vi "Query Sys (To) Parameters (Mode).vi"(8 "error in (no error)":errorcluster, 11 "VISA resource name":refnum<visa-resource-name>) -> (0 "error out":errorcluster, 2 "Mode Parameters":T1={" Mode"=enum."Normal", "Burst #"=-1, "DC Off"=-1, "DC On"=-1, "Period"=nan} {"Period" format="%.6p"}, 3 "VISA resource name out":refnum<visa-resource-name>)   [LabVIEW 2013, in "Berkeley Nucleonics 500 Series.lvlib"]
doc: "This VI is used to read the mode configuration of the system timer (To)."
uses:
  Berkeley Nucleonics 500 Series.lvlib
panel:
  # "Burst"
  # "Duty\nCycle"
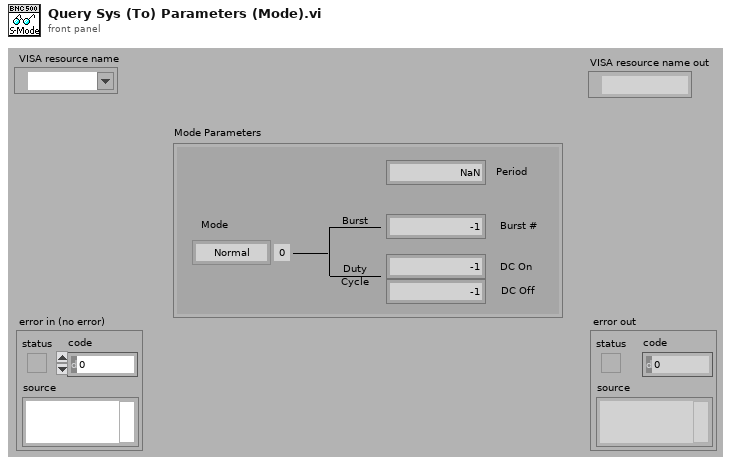
[diagram p1: front panel]
types:
  T1 = cluster{" Mode":enum16{"Normal", "Single", "Burst", "Duty Cycle"}, "Burst #":i32, "DC Off":i32, "DC On":i32, "Period":dbl}
  T2 = cluster{"Sys (To) Mode":enum16{"Normal", "Single", "Burst", "Duty Cycle"}, "Sys (To) Burst #":i32, "Sys (To) DC Off":i32, "Sys (To) DC On":i32, "Sys (To)  Period":dbl}
  T3 = enum16{"Normal", "Single", "Burst", "Duty Cycle"}
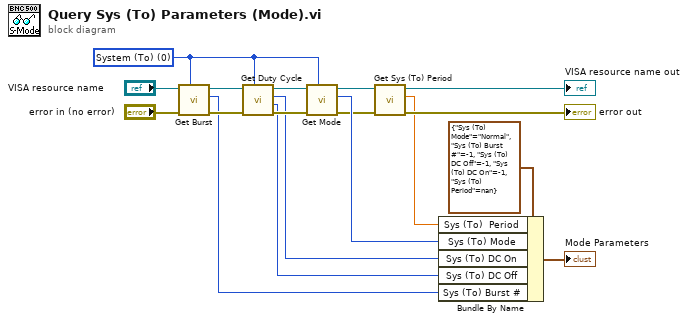
[diagram p0: block diagram]
diagram:
  w6 = 0 items=["System (To)", "Channel A", "Channel B", "Channel C", "Channel D", "Channel E", "Channel F", "Channel G", "Channel H"] ("Channel (1: Chan A)")
  n1 = call "Get Burst.vi"("Channel (1: Chan A)"=w6, "error in (no error)"="error in (no error)", "VISA resource name"="VISA resource name") -> ("error out"=w13:errorcluster, "Burst #"=w11:i32, "VISA resource name out"=w14:refnum<visa-resource-name>)  [unwired: 6 in]
  n2 = call "Get Duty Cycle.vi"("Channel (1: Chan A)"=w6, "error in (no error)"=w13, "VISA resource name"=w14) -> ("error out"=w16:errorcluster, "DC Off"=w10:i32, "DC On"=w9:i32, "VISA resource name out"=w15:refnum<visa-resource-name>)  [unwired: 5 in]
  n3 = call "Get Mode.vi"("Channel (1: Chan A)"=w6, "error in (no error)"=w16, "VISA resource name"=w15) -> ("error out"=w5:errorcluster, "Mode"=w12:T3, "VISA resource name out"=w3:refnum<visa-resource-name>)  [unwired: 6 in]
  n4 = call "Get Sys (To) Period.vi"("error in (no error)"=w5, "VISA resource name"=w3) -> ("error out"=→"error out":errorcluster, "Period"=w1:dbl, "VISA resource name out"=→"VISA resource name out":refnum<visa-resource-name>)  [unwired: 7 in]
  n5 = Bundle By Name(cluster=T2 {"Sys (To) Mode"=enum."Normal", "Sys (To) Burst #"=-1, "Sys (To) DC Off"=-1, "Sys (To) DC On"=-1, "Sys (To)  Period"=nan} ("Mode Parameters"), "Sys (To)  Period"=w1, "Sys (To) Mode"=w12, "Sys (To) DC On"=w9, "Sys (To) DC Off"=w10, "Sys (To) Burst #"=w11) -> (→"Mode Parameters":T2)
